vi "Global_temperature_variables.vi"() -> ()   [LabVIEW 2019]
uses:
  global_temperature_cluster.ctl
panel:
  in  "Temperature-Cluster":T1
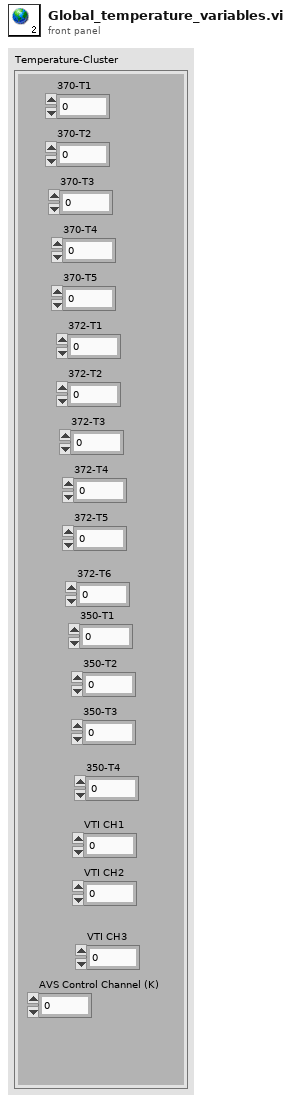
[diagram p1: front panel]
types:
  T1 = typedef "global_temperature_cluster.ctl" = cluster{"370-T1":dbl, "370-T2":dbl, "370-T3":dbl, "370-T4":dbl, "370-T5":dbl, "372-T1":dbl, "372-T2":dbl, "372-T3":dbl, "372-T4":dbl, "372-T5":dbl, "372-T6":dbl, "350-T1":dbl, "350-T2":dbl, "350-T3":dbl, "350-T4":dbl, "VTI CH1":dbl, "VTI CH2":dbl, "VTI CH3":dbl, "AVS Control Channel (K)":dbl}
diagram:
